vi "Mask.vi"(5 "mask key":u32, 6 "error in (no error)":errorcluster, 8 "mask/unmask string in":string) -> (0 "error out":errorcluster, 2 "mask/unmask string out":string)   [LabVIEW 2014, in "FrontPanelPublisher.lvlib" / "Websocket.lvclass"]
uses:
  Websocket.lvclass
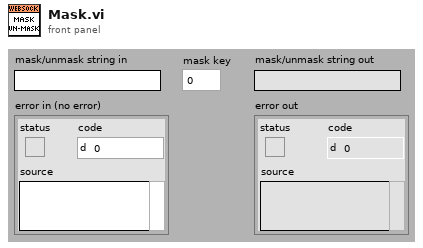
[diagram p1: front panel]
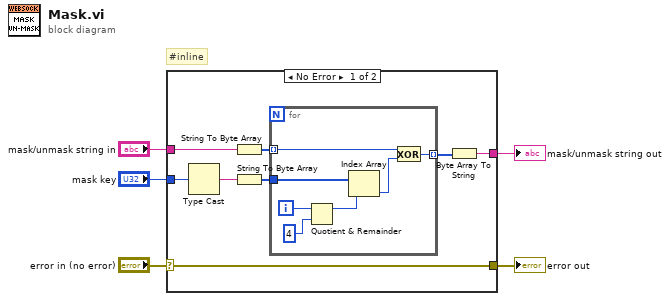
[diagram p0: block diagram]
diagram:
  # "#inline"
  n1 = case shown="No Error" "error in (no error)" {
    selector: "error in (no error)" -> [w6 w21]
    tunnel: "mask/unmask string in" -> [w13 w22]
    tunnel: "mask key" -> [w11 _]
    tunnel: [w7 w22] -> w3
    tunnel: [w6 w21] -> w1
    frame No Error {
      n2 = Type Cast(x=w11) -> (*(type *) &x=w10:string)  [unwired: 1 in]
      n3 = String To Byte Array(string=w13) -> (unsigned byte array=w12:u8[])
      n4 = String To Byte Array(string=w10) -> (unsigned byte array=w9:u8[])
      n5 = for {
        tunnel: w12 -> [w18] mode=indexing
        tunnel: w9 -> [w19]
        tunnel: [w16] -> w8 mode=indexing
        i -> [w20]
        n6 = Quotient & Remainder(x=w20, y=4) -> (x-y*floor(x/y)=w14:i32)  [unwired: 1 out]
        n7 = Index Array(array=w19, index=w14) -> (element=w17:u8)
        n8 = Exclusive Or(1:w17, 2:w18) -> (0:w16:u8)
      }
      n9 = Byte Array To String(unsigned byte array=w8) -> (string=w7:string)
    }
    frame Error {
    }
  }
  "mask/unmask string out" <- w3
  "error out" <- w1
